vi "Initialise.vi"(10 "Size":u16 format="%04x", 11 "Base Address":u16 format="%04x") -> (3 "EEPROM out":refnum<class "RAM.lvclass">)   [LabVIEW 2021, in "RAM.lvclass"]
uses:
  RAM.lvclass
  RAM.lvclass/RAM.ctl
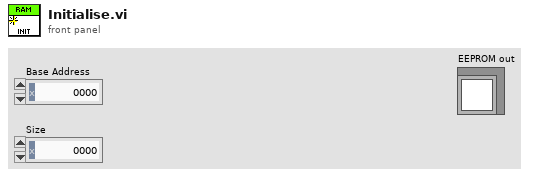
[diagram p1: front panel]
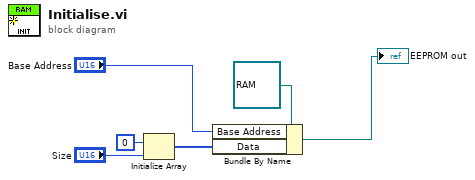
[diagram p0: block diagram]
diagram:
  n1 = Initialize Array(u8 0 ("element"), "Size") -> (w4:u8[])
  n2 = Bundle By Name(cluster=refnum<class "RAM.lvclass"> refnum ("EEPROM in"), "Base Address"="Base Address", "Data"=w4) -> (→"EEPROM out":refnum<class "RAM.lvclass">)
